vi "destroyAll.vi"(8 "error in (no error)":errorcluster, 11 "SAL_Events in":refnum<class "SAL_Events.lvclass">) -> (0 "error out":errorcluster, 3 "SAL_Events out":refnum<class "SAL_Events.lvclass">)   [LabVIEW 2016, in "SAL_Events.lvclass"]
uses:
  SAL_Events.lvclass
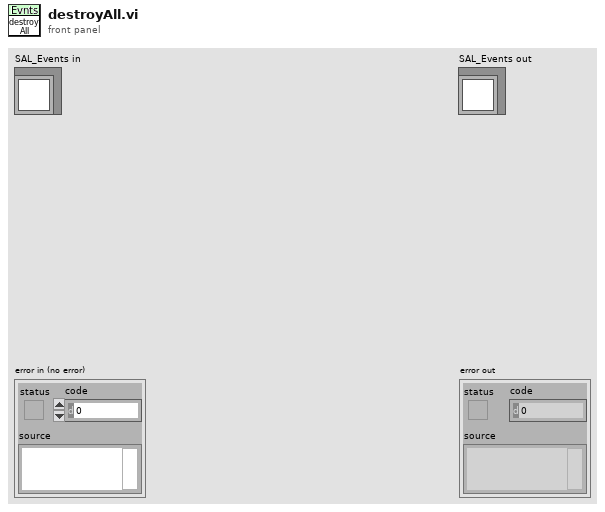
[diagram p1: front panel]
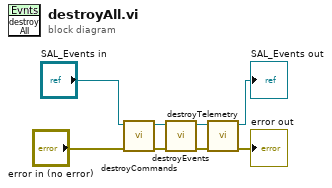
[diagram p0: block diagram]
diagram:
  n1 = call "destroyCommands.vi"("error in (no error)"="error in (no error)", "SAL_Events in"="SAL_Events in") -> ("error out"=w2:errorcluster, "SAL_Events out"=w4:refnum<class "SAL_Events.lvclass">)  [unwired: 8 in]
  n2 = call "destroyEvents.vi"("error in (no error)"=w2, "SAL_Events in"=w4) -> ("error out"=w1:errorcluster, "SAL_Events out"=w3:refnum<class "SAL_Events.lvclass">)  [unwired: 8 in]
  n3 = call "destroyTelemetry.vi"("error in (no error)"=w1, "SAL_Events in"=w3) -> ("error out"=→"error out":errorcluster, "SAL_Events out"=→"SAL_Events out":refnum<class "SAL_Events.lvclass">)  [unwired: 8 in]
